vi "DAC Init Results.vi"(8 "error in":errorcluster, 9 "Log Details?":bool, 10 "tdms file":refnum<k34>, 11 "DAC Inclino in":refnum<class "DAC Inclinometer.lvclass">) -> (0 "error out":errorcluster, 2 "tdms file out":refnum<k34>)   [LabVIEW 2019, in "DAC.lvlib" / "DAC Inclinometer.lvclass"]
uses:
  DAC Inclinometer.lvclass
  DAC.lvclass
  C:/Users/wg/Documents/LV_Projects/test-stand/App/DAC/DAC.lvclass
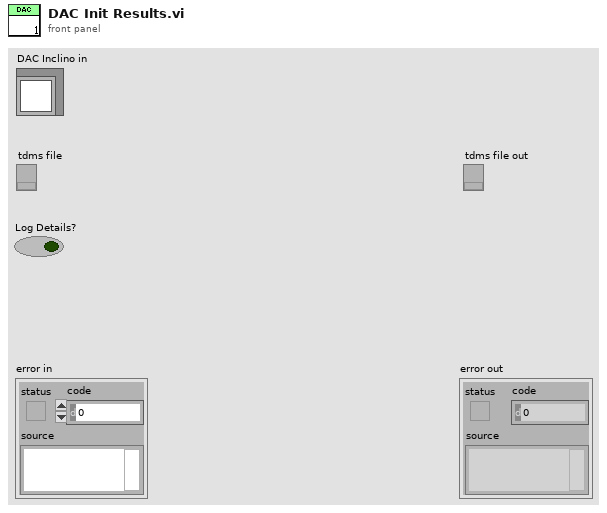
[diagram p1: front panel]
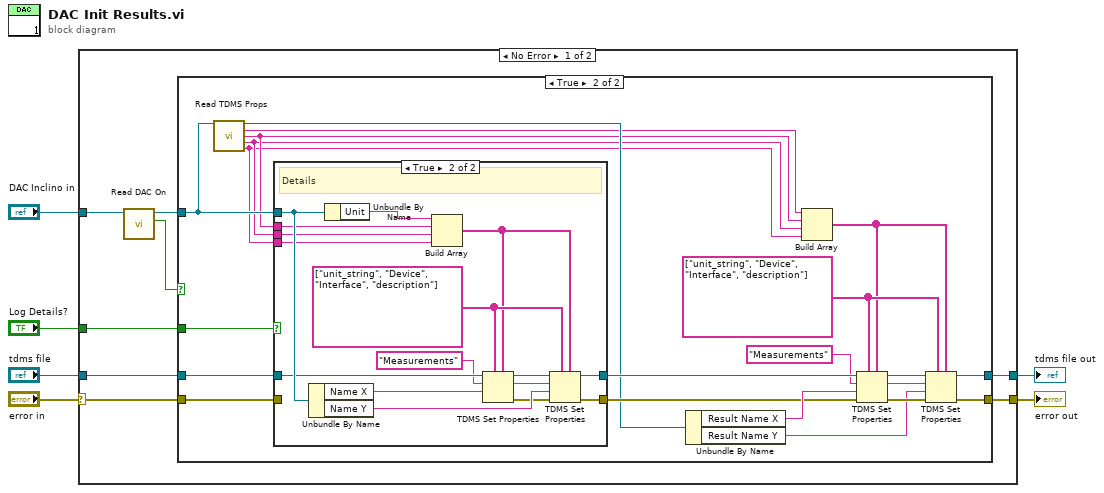
[diagram p0: block diagram]
diagram:
  n1 = case shown="No Error" "error in" {
    selector: "error in" -> [w7 w57]
    tunnel: [w9 w57] -> w6
    tunnel: "DAC Inclino in" -> [w8 _]
    tunnel: "tdms file" -> [w12 w56]
    tunnel: [w10 w56] -> w5
    tunnel: "Log Details?" -> [w11 _]
    frame No Error {
      n2 = call "Read DAC On.vi"("DAC in"=w8) -> ("DAC On"=w13:bool, "DAC out"=w14:refnum<class "DAC Inclinometer.lvclass">)  [unwired: 8 in, 1 out]
      n3 = case shown="True" w13 {
        tunnel: w12 -> [w16 w35]
        tunnel: [w16 w26] -> w10
        tunnel: [w15 w25] -> w9
        tunnel: w14 -> [_ w22]
        tunnel: w11 -> [_ w36]
        tunnel: w7 -> [w15 w23]
        frame False {
        }
        frame True {
          w29 = string[] ["unit_string", "Device", "Interface", "description"] ("property names")
          n4 = call "Read TDMS Props.vi"("DAC in"=w22) -> ("DAC out"=w21:refnum<class "DAC Inclinometer.lvclass">, "Result Unit"=w20:string, "DAC Device"=w19:string, "DAC IO"=w18:string, "DAC Description"=w17:string)  [unwired: 10 in]
          n5 = case shown="True" w36 {
            tunnel: w35 -> [w39 w52]
            tunnel: [w39 w44] -> w33
            tunnel: [w38 w45] -> w34
            tunnel: w22 -> [_ w54]
            tunnel: w23 -> [w38 _]
            tunnel: w19 -> [_ w42]
            tunnel: w18 -> [_ w41]
            tunnel: w17 -> [_ w40]
            frame False {
            }
            frame True {
              w49 = string[] ["unit_string", "Device", "Interface", "description"] ("property names")
              # "Details"
              n6 = Unbundle By Name(w54) -> ("Name X"=w53:string, "Name Y"=w47:string)
              n7 = Unbundle By Name(w54) -> ("Unit"=w55:string)
              n8 = Build Array(w55, w42, w41, w40) -> (w48:string[])
              n9 = TDMS Set Properties(5:w48, 7:w49, 9:w53, 10:"Measurements" ("group name in (Untitled)"), 11:w52) -> (0:w46:errorcluster, 2:w43:string, 3:w51:refnum<k34>)  [unwired: 1 in, 1 out]
              n10 = TDMS Set Properties(5:w48, 7:w49, 8:w46, 9:w47, 10:w43, 11:w51) -> (0:w45:errorcluster, 3:w44:refnum<k34>)  [unwired: 2 out]
            }
          }
          n11 = Unbundle By Name(w21) -> ("Result Name X"=w37:string, "Result Name Y"=w27:string)
          n12 = Build Array(w20, w19, w18, w17) -> (w28:string[])
          n13 = TDMS Set Properties(5:w28, 7:w29, 8:w34, 9:w37, 10:"Measurements" ("group name in (Untitled)"), 11:w33) -> (0:w31:errorcluster, 2:w24:string, 3:w32:refnum<k34>)  [unwired: 1 out]
          n14 = TDMS Set Properties(5:w28, 7:w29, 8:w31, 9:w27, 10:w24, 11:w32) -> (0:w25:errorcluster, 3:w26:refnum<k34>)  [unwired: 2 out]
        }
      }
    }
    frame Error {
    }
  }
  "error out" <- w6
  "tdms file out" <- w5
